vi "Access Module Limits.vi"(8 "error in":errorcluster, 11 "3300 in":refnum<class "3300.lvclass">) -> (0 "error out":errorcluster, 2 "Limits":dbl[](array[numeric]), 3 "3300 out":refnum<class "3300.lvclass">)   [LabVIEW 2019, in "3300.lvlib" / "3300.lvclass"]
uses:
  Library/3300.lvclass
  C:/Users/Public/Documents/Development/builds/Instruments/Electronic Load.lvlibp/Library/Electronic Load.lvclass
  builds/Instruments/Electronic Load.lvlibp/Accessors/Settings/Read Mode.vi
  Accessors/Read Active Module.vi
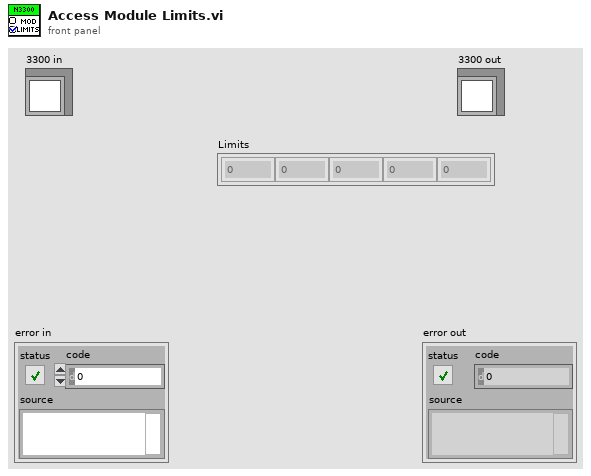
[diagram p1: front panel]
types:
  T1 = typedef "Electronic Load.lvlibp/Electronic Load.lvclass/E-Load Mode.ctl" = enum16{"Current", "Resistance", "Voltage"}
  T2 = typedef "3300.lvlib/3300.lvclass/Modules.ctl" = enum16{"N3302A", "N3303A", "N3304A", "N3305A", "N3306A", "N3307A"}
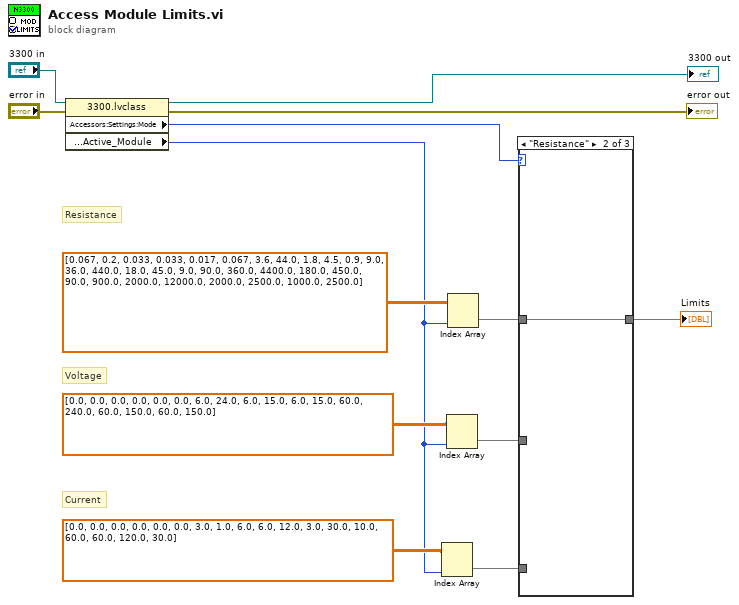
[diagram p0: block diagram]
diagram:
  # "Current"
  # "Voltage"
  # "Resistance"
  n1 = property class="3300.lvclass"(reference="3300 in", error in="error in") -> (reference out=→"3300 out":refnum<class "3300.lvclass">, error out=→"error out":errorcluster, "Accessors:Settings:Mode"=w6:T1, "Private:Accessors:Active_Module"=w1:T2)
  n2 = Index Array(array=dbl[][] [[0.0, 0.0, 0.0, 0.0, 0.0, 0.0], [3.0, 1.0, 6.0, 6.0, 12.0, 3.0], [30.0, 10.0, 60.0, 60.0, 120.0, 30.0]], index (col)=w1) -> (element=w3:dbl[])  [unwired: 1 in]
  n3 = Index Array(array=dbl[][] [[0.0, 0.0, 0.0, 0.0, 0.0, 0.0], [6.0, 24.0, 6.0, 15.0, 6.0, 15.0], [60.0, 240.0, 60.0, 150.0, 60.0, 150.0]], index (col)=w1) -> (element=w2:dbl[])  [unwired: 1 in]
  n4 = Index Array(array=dbl[][] [[0.067, 0.2, 0.033, 0.033, 0.017, 0.067], [3.6, 44.0, 1.8, 4.5, 0.9, 9.0], [36.0, 440.0, 18.0, 45.0, 9.0, 90.0], [360.0, 4400.0, 180.0, 450.0, 90.0, 900.0], [2000.0, 12000.0, 2000.0, 2500.0, 1000.0, 2500.0]], index (col)=w1) -> (element=w5:dbl[])  [unwired: 1 in]
  n5 = case shown="\"Resistance\"" w6 {
    tunnel: [w14 w15 w16] -> w4
    tunnel: w5 -> [_ w15 _]
    tunnel: w3 -> [w14 _ _]
    tunnel: w2 -> [_ _ w16]
    frame "Current", Default {
    }
    frame "Resistance" {
    }
    frame "Voltage" {
    }
  }
  "Limits" <- w4
